vi "get_device_attribute.vi"(6 "timeout (ms)":i32=10000, 7 "IP address":string, 8 "error in (no error)":errorcluster, 9 "token cluster in":T1, 10 "Attribute name":string, 11 "client handle":T2) -> (0 "error out":errorcluster, 1 "token cluster":T1, 2 "Attribute value":string, 3 "client handle out":T2)   [LabVIEW 2018]
uses:
  <vilib>/httpClient/ClientHandle.ctl
  <vilib>/httpClient/LabVIEWHTTPClient.lvlib
panel:
  out "headers":string
  out "status code":string
  out "msg":string
  out "reponse":string
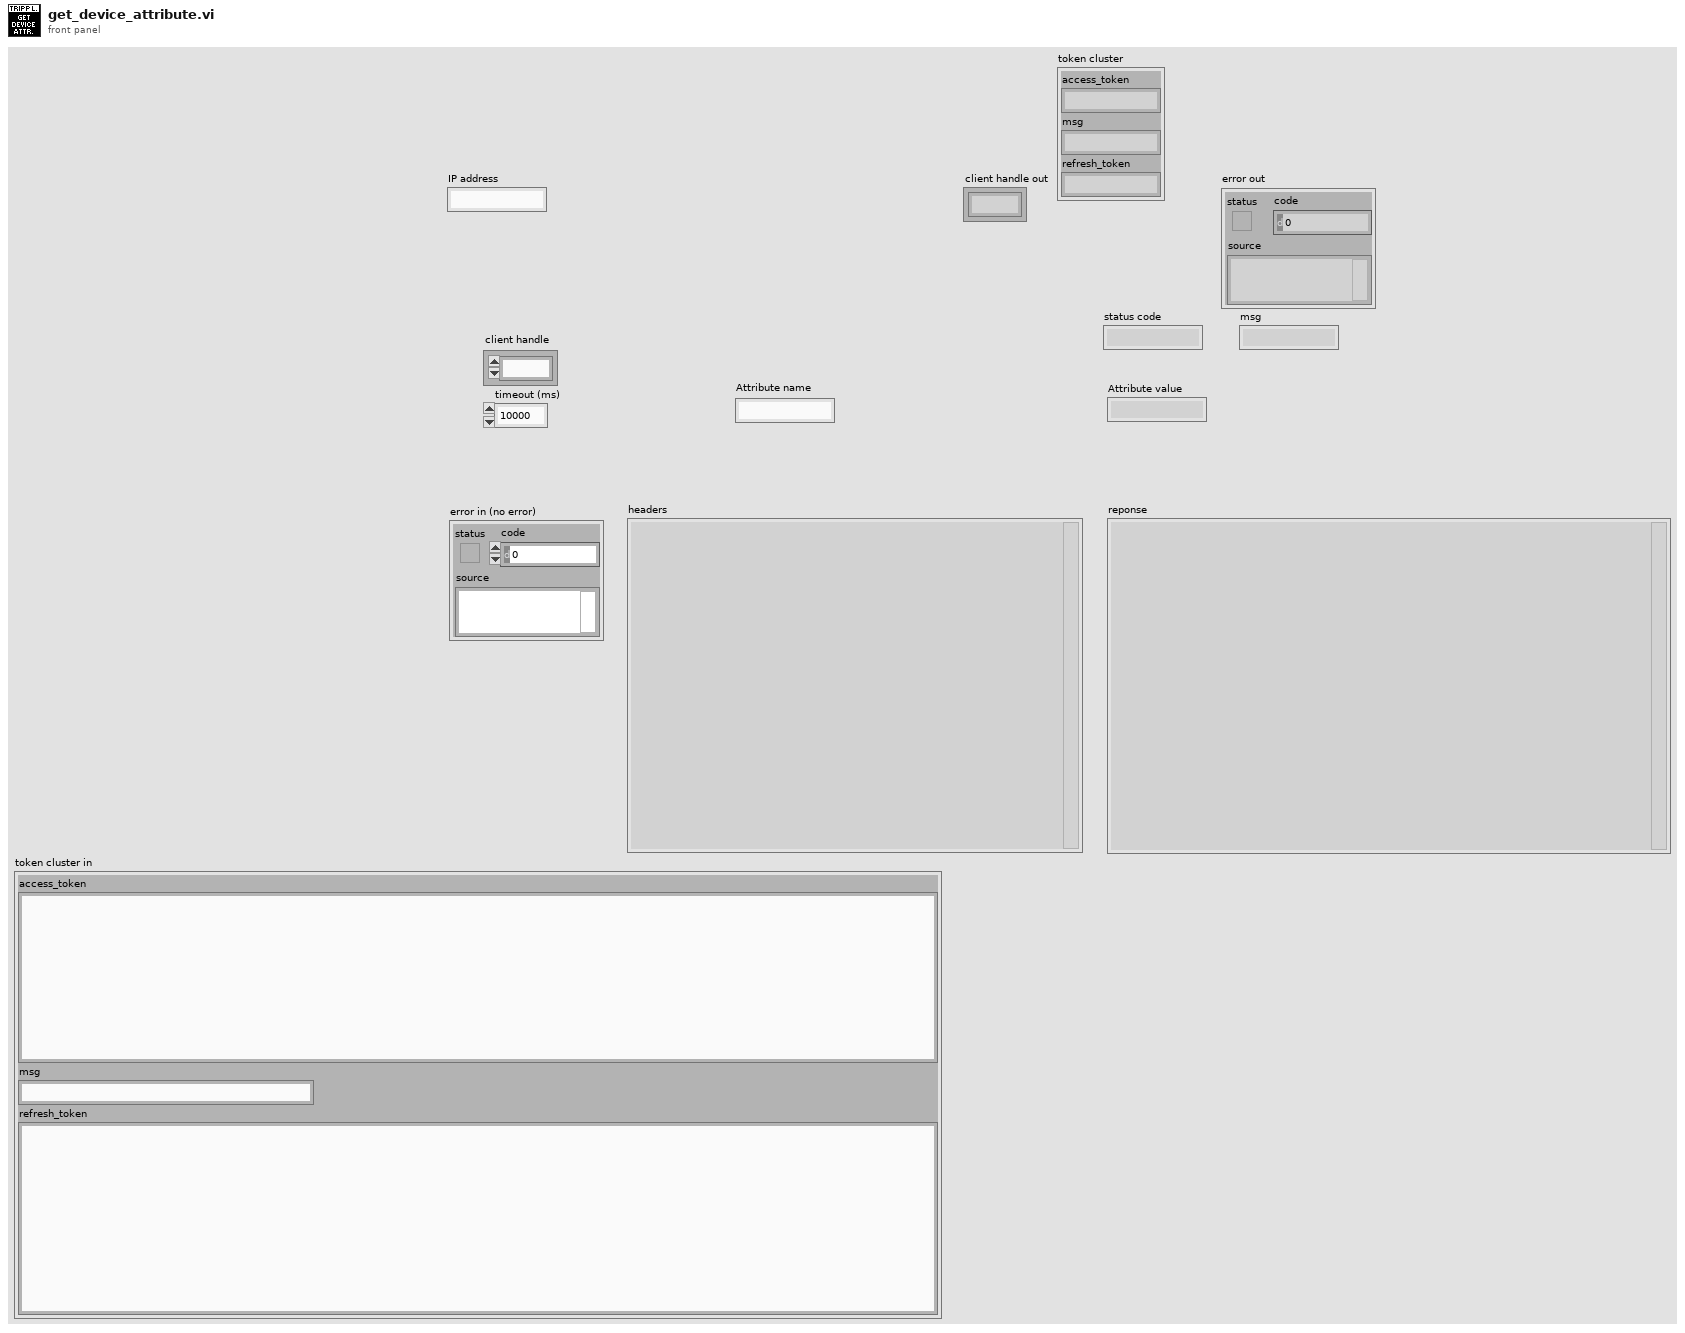
[diagram p1: front panel]
types:
  T1 = cluster{"access_token":string, "msg":string, "refresh_token":string}
  T2 = typedef "LabVIEWHTTPClient.lvlib/ClientHandle.ctl" = refnum<k1>
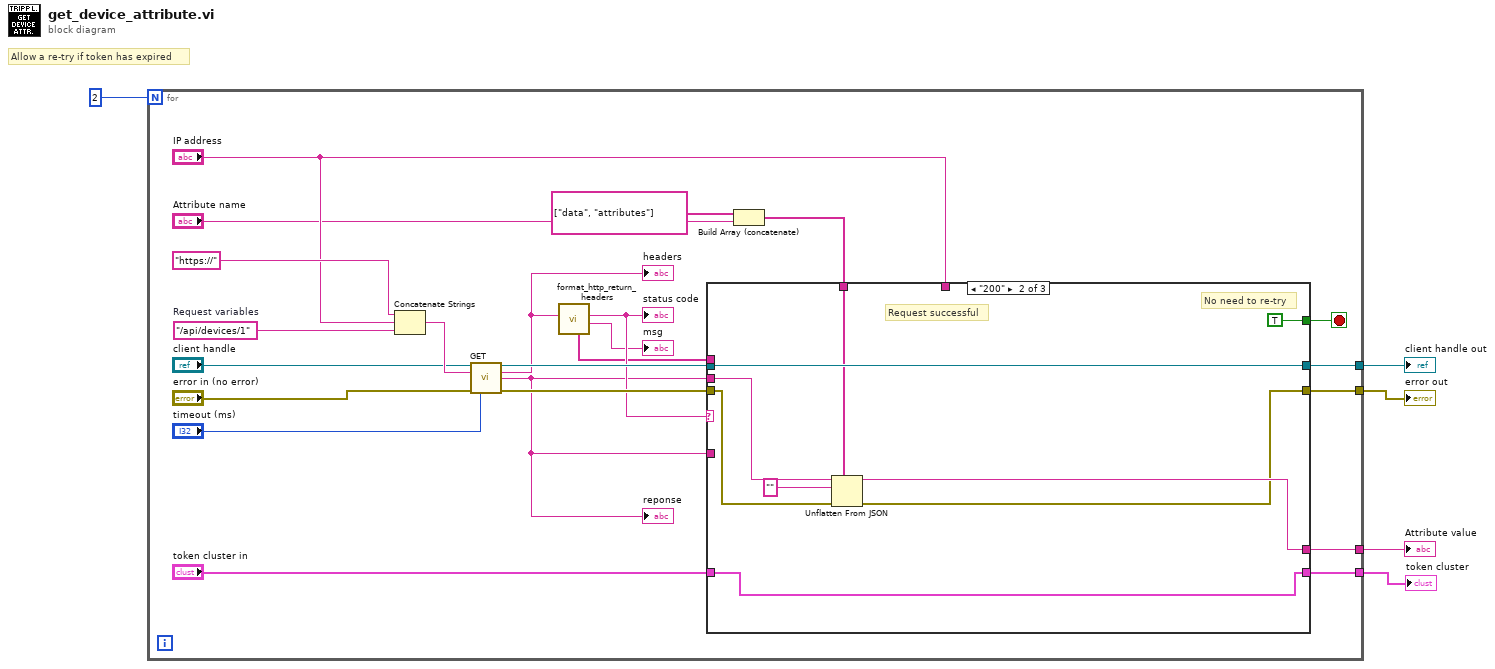
[diagram p0: block diagram]
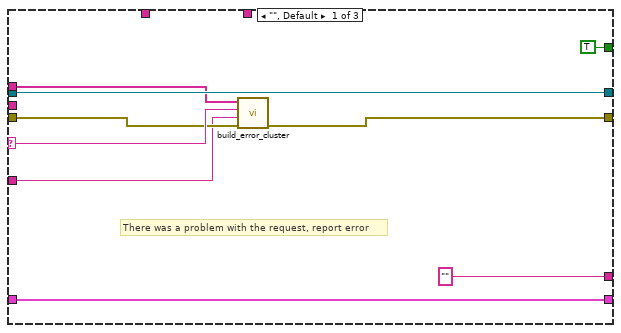
[diagram p2: hidden frame]
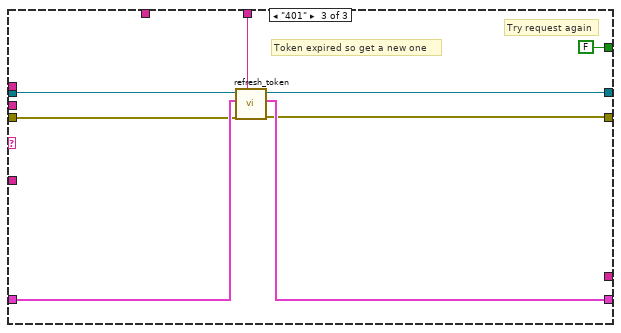
[diagram p3: hidden frame]
diagram:
  # "Allow a re-try if token has expired"
  n1 = for {
    N: 2 -> [_]
    tunnel: [w23] -> w5
    tunnel: [w22] -> w4
    tunnel: [w14] -> w3
    tunnel: [w11] -> w2
    stop <- w9 stop-if-true
    w25 = "/api/devices/1"  # Request variables
    n2 = Concatenate Strings("https://", "IP address", w25) -> (w28:string)
    n3 = call <vilib>:"GET.vi"("client handle"="client handle", "url"=w28, "error in (no error)"="error in (no error)", "timeout (10000)"="timeout (ms)") -> ("client handle out"=w26:T2, "headers"=w21:string, "body"=w13:string, "error out"=w27:errorcluster)  [unwired: 8 in]
    "reponse" <- w13
    "headers" <- w21
    n4 = call "format_http_return_headers.vi"("headers in"=w21) -> ("msg"=→"msg":string, "status code"=w20:string, "headers array"=w18:string[])  [unwired: 8 in]
    "status code" <- w20
    n5 = Build Array (concatenate)(string[] ["data", "attributes"], "Attribute name") -> (w6:string[])
    n6 = case shown="\"200\"" w20 {
      selector: w20 -> [w36 _ _]
      tunnel: w27 -> [w34 w45 w50]
      tunnel: w13 -> [_ w43 _]
      tunnel: w26 -> [w37 w46 w52]
      tunnel: [w33 w39 w49] -> w23
      tunnel: [w37 w46 w51] -> w22
      tunnel: ["" ("body") w40 _] -> w14
      tunnel: w18 -> [w35 _ _]
      tunnel: w13 -> [w31 _ _]
      tunnel: "token cluster in" -> [w30 w42 w54]
      tunnel: [w30 w42 w53] -> w11
      tunnel: "IP address" -> [_ _ w48]
      tunnel: [TRUE TRUE FALSE] -> w9
      tunnel: w6 -> [_ w38 _]
      frame "", Default {
        # "There was a problem with the request, report error"
        n7 = call "build_error_cluster.vi"("error in (no error)"=w34, "error msg (JSON)"=w31, "status code"=w36, "headers array"=w35) -> ("error out"=w33:errorcluster)  [unwired: 7 in]
      }
      frame "200" {
        # "No need to re-try"
        # "Request successful"
        n8 = Unflatten From JSON(path=w38, JSON string=w43, type and defaults="", error in (no error)=w45) -> (value=w40:string, error out=w39:errorcluster)  [unwired: 3 in]
      }
      frame "401" {
        # "Try request again"
        # "Token expired so get a new one"
        n9 = call "refresh_token.vi"("IP address"=w48, "error in (no error)"=w50, "token cluster in"=w54, "client handle"=w52) -> ("error out"=w49:errorcluster, "token cluster"=w53:T1, "client handle out"=w51:T2)  [unwired: 5 in]
      }
    }
  }
  "error out" <- w5
  "client handle out" <- w4
  "Attribute value" <- w3
  "token cluster" <- w2
